vi "communicateWebServices.vi"(8 "ErrorIn":errorcluster, 11 "QueuesIn":T1) -> (0 "ErrorOut":errorcluster, 3 "QueuesOut":T1)   [LabVIEW 2019]
uses:
  utilities/AQueues.ctl
  UIVIs/AccelerationDataFrames.ctl
  AmasterVIs/ACommand.ctl
  communicateWebServicesVIs/CommunicateWebServicesState.ctl
  communicateWebServicesVIs/WebServicesData.ctl
  UIVIs/UIOutput.ctl
  AmasterVIs/AThreads.ctl
  <vilib>/dex/Stream Element Allocation Mode.ctl
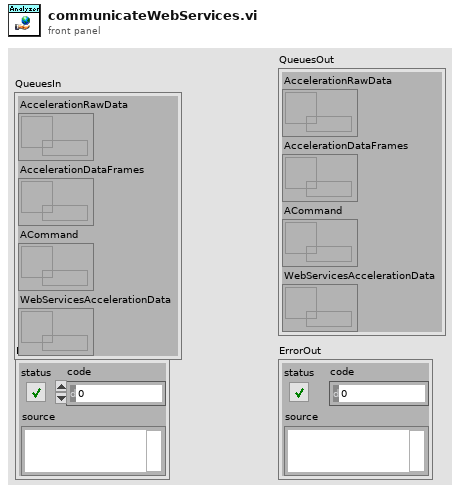
[diagram p1: front panel]
types:
  T1 = typedef "AQueues.ctl" = cluster{"AccelerationRawData":refnum<queue>, "AccelerationDataFrames":refnum<queue>, "ACommand":refnum<queue>, "WebServicesAccelerationData":refnum<queue>}
  T2 = typedef "WebServicesData.ctl" = cluster{"AccelerationDataFrames":T3, "UIOutput":T4}
  T3 = typedef "AccelerationDataFrames.ctl" = cluster{"AccelerationData":waveform(dbl)[], "Amplitudes":cluster{"f0":dbl, "df":dbl, "real part":dbl[]}[], "Phases":cluster{"f0":dbl, "df":dbl, "imaginary part":dbl[]}[]}
  T4 = typedef "UIOutput.ctl" = cluster{"Aquiring data":bool, "AnalyzerError":errorcluster, "FIFO overflow":bool, "Analyzing data":bool}
  T5 = typedef "AThreads.ctl" = enum16{"UI", "analyzeAccelerationData", "aquireAccelerationData", "communicateWebServices"}
  T6 = typedef "CommunicateWebServicesState.ctl" = enum16{"Wait for request", "Send data", "End", "Init"}
  T7 = typedef "ACommand.ctl" = enum16{"None", "Start", "Stop", "Restart"}
  T8 = typedef "Stream Element Allocation Mode.ctl" = u32
  T9 = typedef "AnalyzerSettings.ctl" = cluster{"fs [Hz]":dbl, "Create NS Timeout Code":i32, "Destroy NS Timeout Code":i32, "All threads":T5[]}
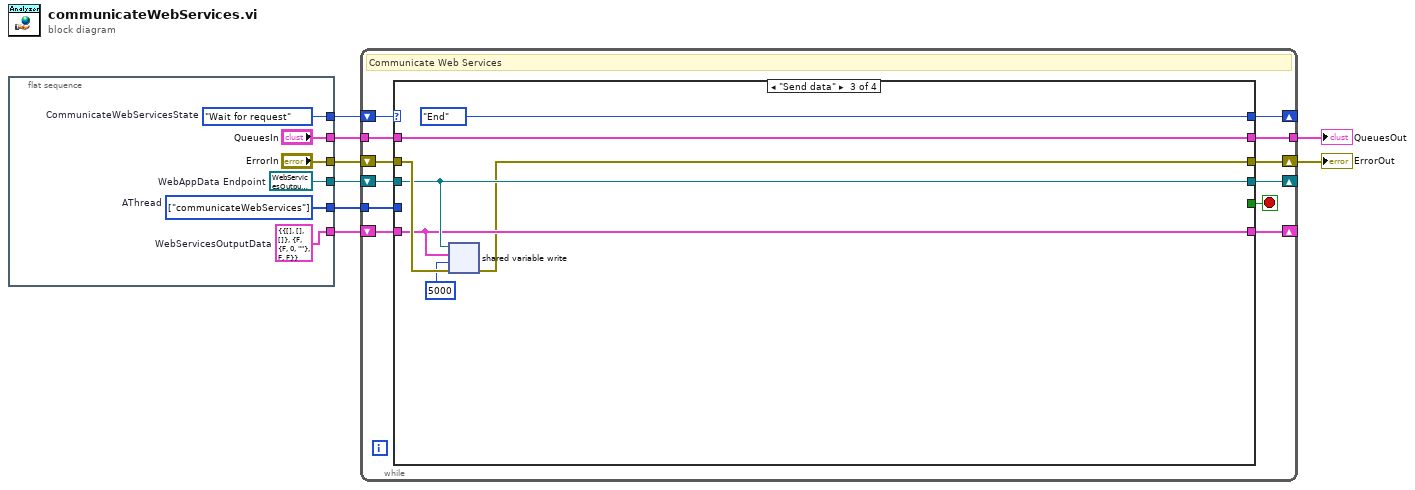
[diagram p0: block diagram]
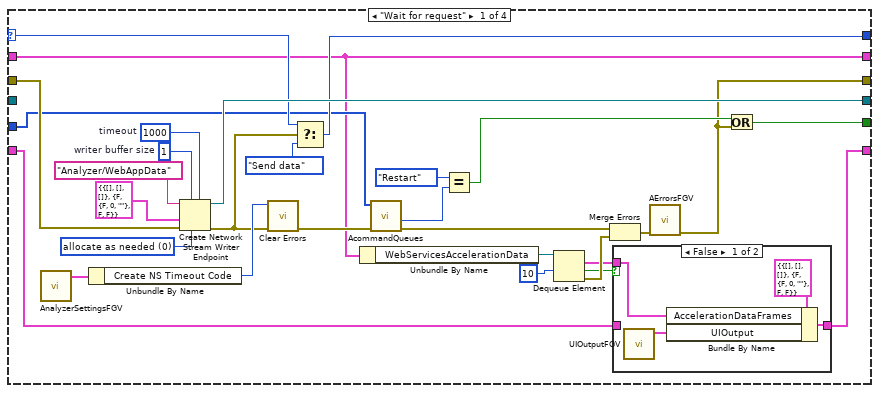
[diagram p2: hidden frame]
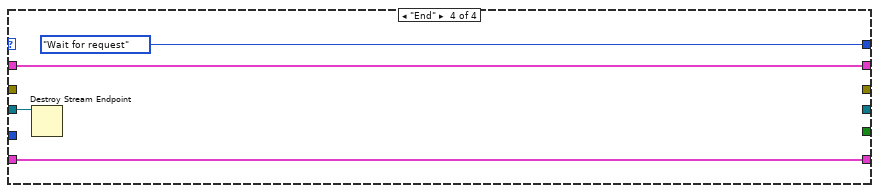
[diagram p5: hidden frame]
diagram:
  n1 = flat-sequence {
    tunnel: [w14] -> w8
    tunnel: ["QueuesIn"] -> w7
    tunnel: ["ErrorIn"] -> w6
    tunnel: [w11] -> w4
    tunnel: [w10] -> w2
    tunnel: [w9] -> w1
    frame #0 {
      w9 = T2 {"AccelerationDataFrames"={"AccelerationData"=[], "Amplitudes"=[], "Phases"=[]}, "UIOutput"={"Aquiring data"=FALSE, "AnalyzerError"={"status"=FALSE, "code"=0, "source"=""}, "FIFO overflow"=FALSE, "Analyzing data"=FALSE}}  # WebServicesOutputData
      w10 = T5[] [enum."communicateWebServices"] items=["UI", "analyzeAccelerationData", "aquireAccelerationData", "communicateWebServices"]  # AThread
      w11 = refnum<k21> refnum  # WebAppData Endpoint
      w14 = CommunicateWebServicesState."Wait for request"  # CommunicateWebServicesState
    }
  }
  n2 = while {
    shift-right: [w23] -> _
    shift-left: w8 -> [w26]
    tunnel: w7 -> [w25]
    shift-right: [w19] -> w5
    shift-left: w6 -> [w24]
    shift-right: [w21] -> _
    shift-left: w4 -> [w22]
    tunnel: [w18] -> w3
    tunnel: w2 -> [w17]
    shift-right: [w15] -> _
    shift-left: w1 -> [w16]
    stop <- w20 stop-if-true
    # "Communicate Web Services"
    n3 = case shown="\"Send data\"" w26 {
      selector: w26 -> [w45 _ _ _]
      tunnel: w25 -> [w35 w63 w71 w74]
      tunnel: w24 -> [w52 _ w70 _]
      tunnel: [w35 w63 w71 w74] -> w18
      tunnel: [w46 _ CommunicateWebServicesState."End" ("CommunicateWebServicesState") CommunicateWebServicesState."Wait for request" ("CommunicateWebServicesState")] -> w23
      tunnel: [w40 _ w66 _] -> w19
      tunnel: w22 -> [_ w64 w69 w73]
      tunnel: [w50 w64 w69 _] -> w21
      tunnel: [w41 _ _ _] -> w20
      tunnel: w17 -> [w37 _ _ _]
      tunnel: w16 -> [w27 w62 w67 w72]
      tunnel: [w28 w62 w67 w72] -> w15
      frame "Wait for request" {
        w51 = T8 0 items=["allocate as needed", "pre-allocate"] ("element allocation mode")
        w54 = 1000  # timeout
        w55 = 1  # writer buffer size
        n4 = call "AnalyzerSettingsFGV.vi"() -> ("GlobalSettingsOut"=w49:T9)  [unwired: 11 in]
        n5 = Unbundle By Name(w49) -> ("Create NS Timeout Code"=w48:i32)
        n6 = Create Network Stream Writer Endpoint(5:w54, 6:w51, 7:w55, 8:w52, 9:T2 {"AccelerationDataFrames"={"AccelerationData"=[], "Amplitudes"=[], "Phases"=[]}, "UIOutput"={"Aquiring data"=FALSE, "AnalyzerError"={"status"=FALSE, "code"=0, "source"=""}, "FIFO overflow"=FALSE, "Analyzing data"=FALSE}} ("WebServicesOutputData"), 11:"Analyzer/WebAppData" ("writer name")) -> (0:w44:errorcluster, 3:w50:refnum<k21>)  [unwired: 1 in]
        n7 = call <vilib>:"Clear Errors.vi"("error in (no error)"=w44, "specific error code to clear (0: all)"=w48) -> ("error out"=w39:errorcluster)  [unwired: 4 in, 1 out]
        n8 = Select(t=w45, s=w44, f=CommunicateWebServicesState."Send data" ("CommunicateWebServicesState")) -> (s? t:f=w46:T6)
        n9 = Unbundle By Name(w35) -> ("WebServicesAccelerationData"=w34:refnum<queue>)
        n10 = call "AcommandQueues.vi"("ErrorIn"=w39, "AThreads"=w37) -> ("ErrorOut"=w38:errorcluster, "ACommandOut"=w36:T7)  [unwired: 8 in]
        n11 = Equal?(x=ACommand."Restart" ("element"), y=w36) -> (x = y?=w42:bool)
        n12 = Dequeue Element(queue=w34, timeout in ms (-1)=10) -> (element=w29:T3, timed out?=w30:bool, error out=w31:errorcluster)  [unwired: 1 in, 1 out]
        n13 = Merge Errors(w38, w31) -> (w32:errorcluster)
        n14 = case shown="False" w30 {
          tunnel: w29 -> [w58 _]
          tunnel: [w57 w61] -> w28
          tunnel: w27 -> [_ w61]
          frame False {
            n15 = call "UIOutputFGV.vi"() -> ("UIOutputOut"=w59:T4)  [unwired: 10 in, 1 out]
            n16 = Bundle By Name(cluster=T2 {"AccelerationDataFrames"={"AccelerationData"=[], "Amplitudes"=[], "Phases"=[]}, "UIOutput"={"Aquiring data"=FALSE, "AnalyzerError"={"status"=FALSE, "code"=0, "source"=""}, "FIFO overflow"=FALSE, "Analyzing data"=FALSE}} ("WebServicesOutputData"), "AccelerationDataFrames"=w58, "UIOutput"=w59) -> (w57:T2)
          }
          frame True {
          }
        }
        n17 = call "AErrorsFGV.vi"("CriticalErrorIn"=w32) -> ("CriticalErrorOut"=w40:errorcluster)  [unwired: 7 in, 3 out]
        n18 = Or(x=w42, y=w40) -> (x .or. y?=w41:bool)
      }
      frame "Init" {
      }
      frame "Send data" {
        n19 = shared-variable-write(w69, w70, w67, 5000 ("timeout ms (-1)")) -> (w66:errorcluster)  [unwired: 2 out]
      }
      frame "End" {
        n20 = Destroy Stream Endpoint(11:w73) -> ()  [unwired: 1 in, 1 out]
      }
    }
  }
  "ErrorOut" <- w5
  "QueuesOut" <- w3
